vi "读取输入数值类型判断.vi"(8 "error in (no error)":errorcluster caption="错误输入（无错误）", 11 "计算器类输入":refnum<class "计算器类.lvclass">) -> (0 "error out":errorcluster caption="错误输出", 2 "输入数值类型判断":bool, 3 "计算器类输出":refnum<class "计算器类.lvclass">)   [LabVIEW 2020, in "计算器类.lvclass"]
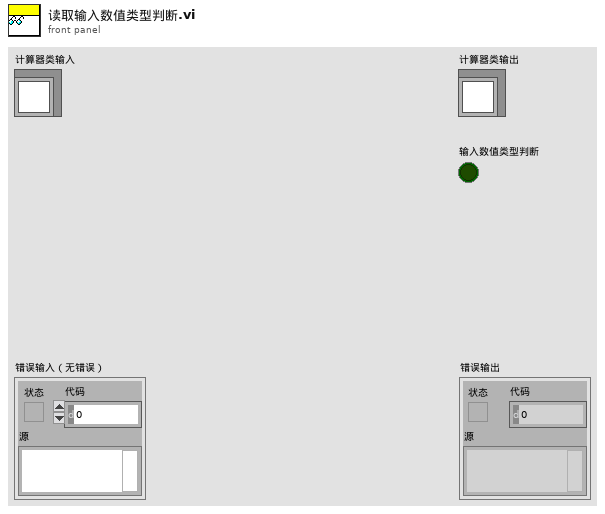
[diagram p1: front panel]
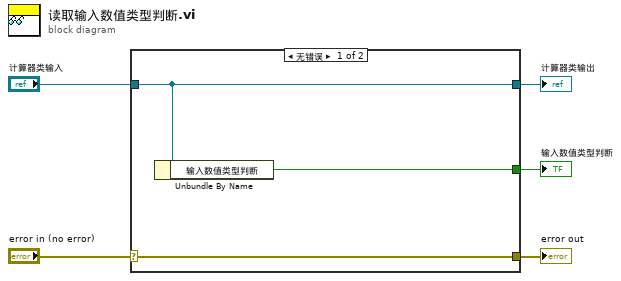
[diagram p0: block diagram]
diagram:
  n1 = case shown="无错误" "error in (no error)" {
    selector: "error in (no error)" -> [w8 w9]
    tunnel: [w8 w9] -> w4
    tunnel: [w7 w10] -> w2
    tunnel: "计算器类输入" -> [w7 w10]
    tunnel: [w6 _] -> w1
    frame No Error {
      n2 = Unbundle By Name(w7) -> ("输入数值类型判断"=w6:bool)
    }
    frame Error {
    }
  }
  "error out" <- w4
  "计算器类输出" <- w2
  "输入数值类型判断" <- w1
